vi "Calc Init.vi"(8 "error in (no error)":errorcluster, 10 "Config":refnum<class "Channel Config.lvclass">, 11 "Min Calc in":refnum<class "Min Calc.lvclass">) -> (0 "error out":errorcluster, 3 "Min Calc out":refnum<class "Min Calc.lvclass">)   [LabVIEW 2020, in "VolatusCalcs.lvlib" / "Min Calc.lvclass"]
uses:
  Min Calc.lvclass
  Min Calc.lvclass/Min Calc.ctl
  lv-cdm/CDM-Config/Config Element/Config Element.lvclass
  VolatusConfig/VolatusConfigElement/VolatusConfigElement.lvclass
  VolatusConfig/Channel/Channel Config.lvclass
  C:/dev/lv20CE/relink/lv-volatus/VolatusConfig/VolatusConfigElement/VolatusConfigElement.lvclass
  C:/dev/lv20CE/relink/lv-volatus/VolatusConfig/Channel/Channel Config.lvclass
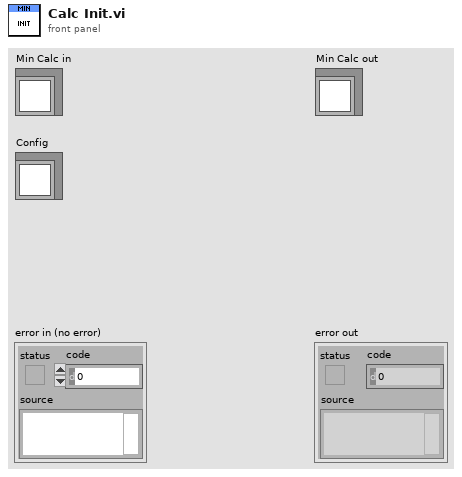
[diagram p1: front panel]
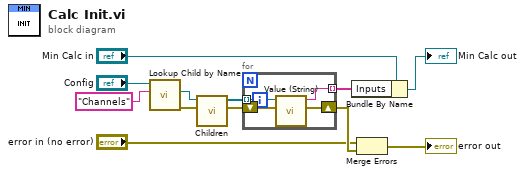
[diagram p0: block diagram]
diagram:
  n1 = call "Lookup Child by Name.vi"("Child Name"="Channels", "VolatusConfigElement in"="Config") -> ("error out"=w11:errorcluster, "Child"=w10:refnum<class "Config Element.lvclass">)  [unwired: 6 in, 2 out]
  n2 = call "Children.vi"("error in (no error)"=w11, "Config Element in"=w10) -> ("error out"=w9:errorcluster, "Elements"=w8:refnum<class "Config Element.lvclass">[])  [unwired: 8 in]
  n3 = for {
    shift-right: [w14] -> w6
    shift-left: w9 -> [w16]
    tunnel: w8 -> [w15] mode=indexing
    tunnel: [w13] -> w7 mode=indexing
    n4 = call "Value (String).vi"("error in (no error)"=w16, "Config Element in"=w15) -> ("error out"=w14:errorcluster, "String Value"=w13:string)  [unwired: 8 in]
  }
  n5 = Bundle By Name(cluster="Min Calc in", "Inputs"=w7) -> (→"Min Calc out":refnum<class "Min Calc.lvclass">)
  n6 = Merge Errors("error in (no error)", w6) -> (→"error out":errorcluster)
